vi "Set Camera Configuration.vi"(8 "error in (no error)":errorcluster, 11 "CCDCamera in":refnum<class "Simulated_CCD_Camera.lvclass">) -> (0 "error out":errorcluster, 3 "CCDCamera out":refnum<class "Simulated_CCD_Camera.lvclass">)   [LabVIEW 2018, in "Simulated_CCD_Camera.lvclass"]
uses:
  Simulated_CCD_Camera.lvclass
  Simulated_CCD_Camera.lvclass/Simulated_CCD_Camera.ctl
  Interface/Interface.lvclass/Interface.ctl
  Interface/Interface.lvclass
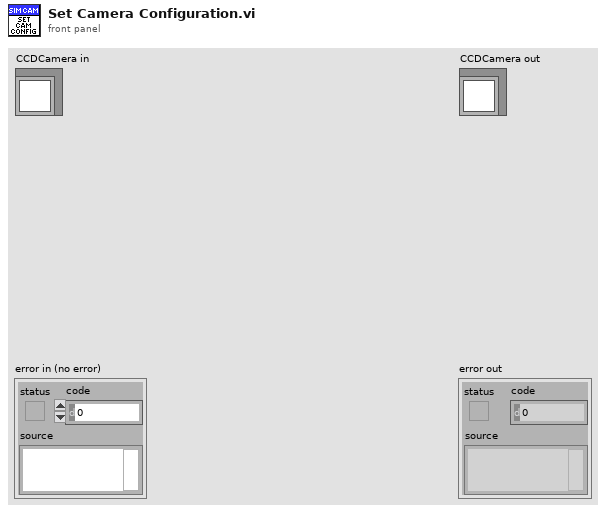
[diagram p1: front panel]
types:
  T1 = cluster{"PREAMP":u16, "READOUT_RATE":u16, "EM_GAIN":u16, "VBIN":u16, "INITIAL_LINE":u16, "INITIAL_COLUMN":u16, "FINAL_LINE":u16, "FINAL_COLUMN":u16, "TRIGGER_MODE":u16, "HBIN":u16, "SHUTTER_TTL":u16, "SHUTTER_MODE":u16, "SHUTTER_OPENING_TIME":u16, "SHUTTER_CLOSING_TIME":u16, "VERTICAL_SHIFT_SPEED":u16, "READ_MODE":u16, "FRAME_TRANSFER":bool, "VERTICAL_CLOCK_VOLTAGE":u16, "ACQUISITION_MODE":u16, "AD_CHANNEL":u16, "EM_MODE":u16}
  T2 = cluster{"COOLER_POWER_STATUS":u16, "TEMP":i32, "EXPTIME":dbl, "#FRAMES":u32, "#CUBES":u32}
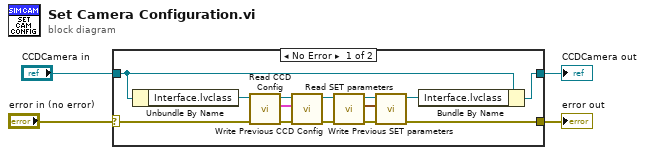
[diagram p0: block diagram]
diagram:
  n1 = case shown="No Error" "error in (no error)" {
    selector: "error in (no error)" -> [w17 w20]
    tunnel: [w11 w20] -> w4
    tunnel: [w5 w19] -> w1
    tunnel: "CCDCamera in" -> [w7 w19]
    frame No Error {
      n2 = Unbundle By Name(w7) -> ("Interface.lvclass"=w18:refnum<class "Interface.lvclass">)
      n3 = call "Read CCD Config.vi"("error in (no error)"=w17, "Interface in"=w18) -> ("error out"=w8:errorcluster, "Previous CCD Config"=w10:T1, "Interface out"=w9:refnum<class "Interface.lvclass">)  [unwired: 7 in]
      n4 = call "Write Previous CCD Config.vi"("error in (no error)"=w8, "Previous CCD Config"=w10, "Interface in"=w9) -> ("error out"=w15:errorcluster, "Interface out"=w16:refnum<class "Interface.lvclass">)  [unwired: 7 in]
      n5 = call "Read SET parameters.vi"("error in (no error)"=w15, "Interface in"=w16) -> ("error out"=w12:errorcluster, "SET parameters"=w14:T2, "Interface out"=w13:refnum<class "Interface.lvclass">)  [unwired: 7 in]
      n6 = call "Write Previous SET parameters.vi"("error in (no error)"=w12, "Previous SET parameters"=w14, "Interface in"=w13) -> ("error out"=w11:errorcluster, "Interface out"=w6:refnum<class "Interface.lvclass">)  [unwired: 7 in]
      n7 = Bundle By Name(cluster=w7, "Interface.lvclass"=w6) -> (w5:refnum<class "Simulated_CCD_Camera.lvclass">)
    }
    frame Error {
    }
  }
  "error out" <- w4
  "CCDCamera out" <- w1
